vi "Gas_Setup.vi"() -> ()   [LabVIEW 2022 SP3]
uses:
  ADAM Controls/Ch_description_ADAM.ctl
  ADAM Controls/Module_type_ADAM.ctl
  ADAM Controls/Function_ADAM.ctl
  ADAM Controls/Channel_State.ctl
  ADAM Controls/Calib_type_ADAM.ctl
  ADAM Controls/Address.ctl
  ADAM Controls/Shut_Off_Valve.ctl
  ADAM Controls/Channel_names.ctl
  Channel_State_Control.ctl
  ADAM Controls/Update_scan_value.ctl
  Anemometry/Anemometry Sub Vis/Globals/Preference_global.vi
panel:
  in  "Change? 2":bool
  out "GMU2 Release Temp Channel":string
  in  "Change?":bool
  out "GMU1 Release Temp Channel":string
  out "Ch names":string[](array[string])
  in  "Select Plug Ins":bool
  in  "Source Info":string[][](table)
  in  "Carrier 1 Very Low":T1
  in  "Carrier 1 Hi-Tec Range":u16(ring) items=["Very Low", "High"]
  in  "Trace Hi-Tec Range":u16(ring) items=["25 ml/min", "300 ml/min"]
  in  "Carrier 1 High":T1
  in  "300 ml/min":T1
  in  "25 ml/min":T1
  in  "Release Orientation":u16(ring) items=["Vertical", "Horizontal 0 Deg", "Downwards", "External System Tests", "Horizontal", "Edit Strings"]
  in  "Source Type":u16(ring) items=["11mm downward facing", "1mm Annulus above tank wall with Internal 2mm Annulus floating roof at 50mm.", "2 x ID=11mm Holes", "23mm IDD=8mm", "2mm Annulus around a quarter of inside of tank wall", "2mm Annulus around inside of tank wall", "4 point source ID=8.5mm located 90 deg apart on 8cm Diameter", "4 x 3mm holes spaced 8mm apart at roof perimeter", "70x70mm", "8  x 3mm holes spaced 10mm apart at roof perimeter", "8mm Annulus around inside of tank wall", "B2 D=6.8mm", "B204 Height 244mm ID 5.5mm", "B230 Height 152.4mm ID 8.5mm", "B30 Area", "B311 ID=11mm", "B331 ID=5.4mm", "B38_8mm_ID_passive", "B38_OD=3.1mm_ID=2mm", "B548 OD=13.8mm ID=3.5mm", "Both_Scrubbers_ID=4mm", "Both_Scrubbers_ID=7mm", "Capped release D=10mm H=10mm Slot=2mm", "D=12mm", "D=13.6mm", "D=16mm (ID=12 mm)", "D=18mm", "D=20mm", "D=22.5mm", "D=3.4mm", "D=5mm (ground release)", "D=6mm (ID=4.2 mm)", "D=7.1mm", "D=9mm", "D=9mm  20mm long passive", "Dext = 8.5 mm", "Exit Port of Solenoid Valve", "H=25:W=100mm", "H=50", "ID=1.6 OD=1.9", "ID=1.9 OD=3.0mm", "ID=103mm", "ID=15 mm 90 deg bend copper tube", "ID=20mm", "ID=24mm", "ID=3.4mm  OD= 4mm", "ID=3.9mm OD=6.3mm", "ID=4.25mm", "ID=4mm", "ID=5.1mm OD=5.8mm (Ground release)", "ID=5.1mm OD=5.8mm (roof release)", "ID=5.1mm at Z= 10mm  (Ground release)", "ID=50mm", "ID=5mm OD=5.8mm", "ID=6mm", "ID=6mm OD=8mm", "ID=7.75mm OD=10mm", "ID=8.6mm", "ID=8mm OD=9mm", "ID=9.2mm", "ID=9.5mm OD=12.5mm", "ID=9mm OD=10mm  Short Passive", "Line Source 100mm  1.07m width", "Line Source 25mm  1.3m long  perp to flow", "Line Source 25x1300", "Line Source 50mm  1.07m Wide", "Line source parallel to flow", "None", "Permeability_rig", "Pond_No1&2_140mm", "Pond_No1&2_84mm", "Pond_No1_84mm", "Pond_No2_84mm", "ROSE 9mm at last grid", "SAV ID=3.5mm", "Sample tubes in source", "Single 5mm Stack", "Single 7.9 mm stack", "THORP  ID=5.1mm", "Twin 5mm Stacks", "Twin Passive Stacks ID=8mm OD=8.7mm", "UKAEA ID=1.7mm", "W=50mm", "Edit Strings"]
  in  "Gas Remaining":string[][](table)
  in  "Carrier 2 Gas":u16(ring) items=["Air", "Nitrogen", "Helium", "CO2", "Krypton", "None"]
  in  "Trace Gas":u16(ring) items=["Propane", "Ethane"]
  in  "Carrier 1 Gas":u16(ring) items=["Air", "Nitrogen", "Helium", "CO2", "Krypton", "None"]
  out "Numerical Values":dbl[](array[numeric]) format="%.9f"
  out "Ch Description Array":T2[](array[typedef]) {"Duty" format="%016b"; "D" format="%#_5g"; "C" format="%#_5g"; "B" format="%#_5g"; "A" format="%#_5g"}
  out "dup reference":refnum<vi>
  in  "stop":bool
  in  "OK":bool
  # "50l/min"
  # "50l/min"
  # "700l/min"
  # "50\nml/min"
  # "300\nml/min"
  # "5l/min"
  # "25\nml/min\nto Source"
  # "Very\nLow\nRange"
  # "High\nRange"
  # "Low\nRange"
  # "To Source"
  # "Dispersion Setup"
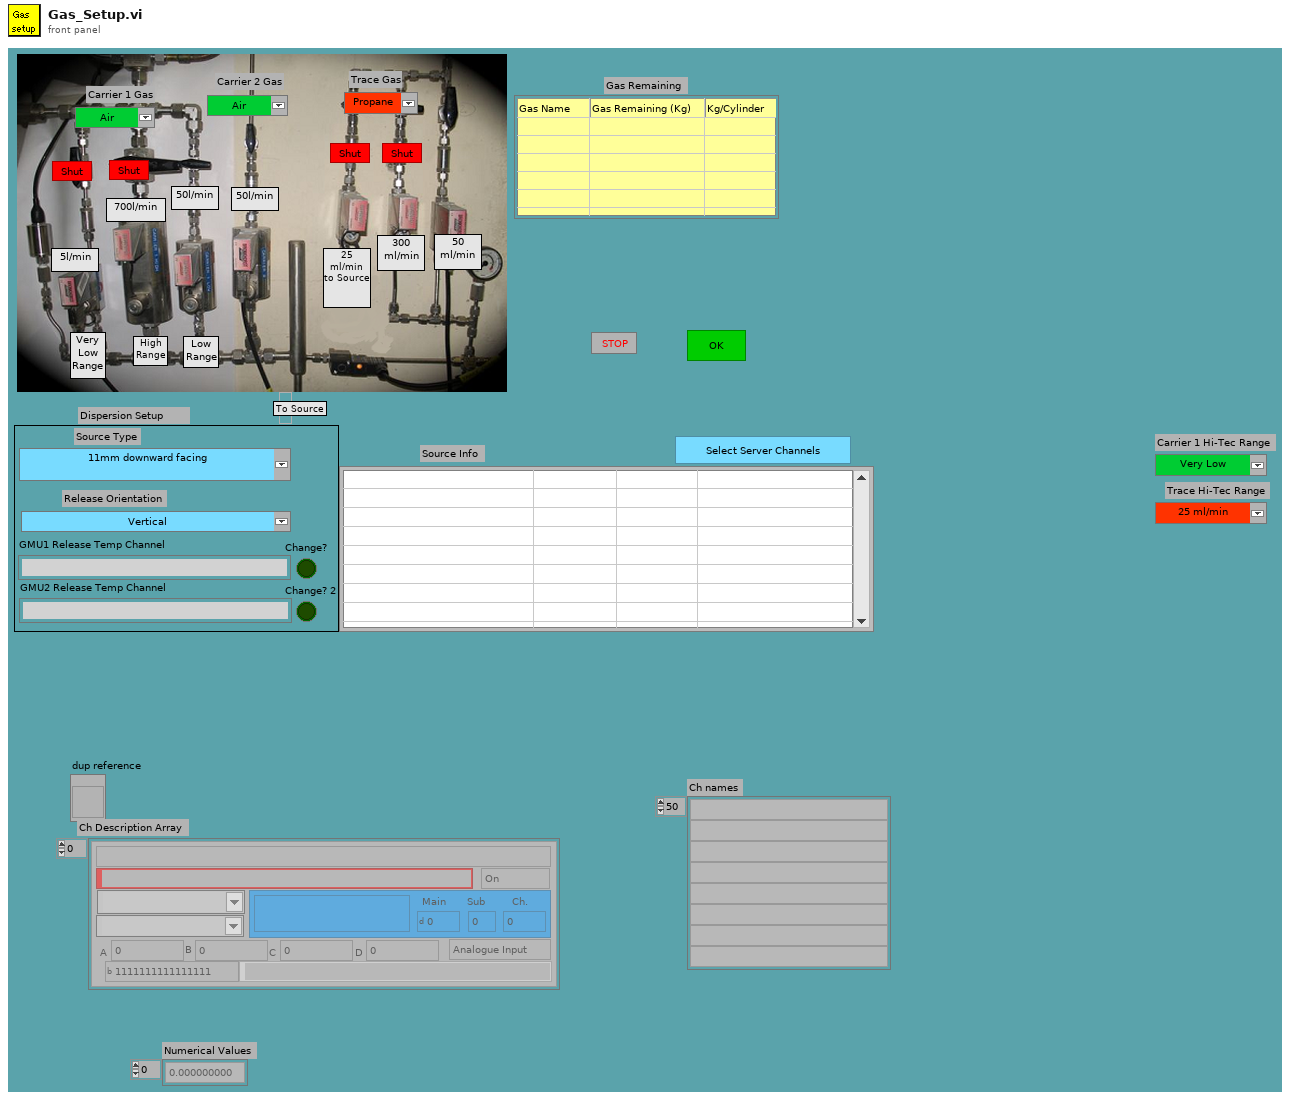
[diagram p1: front panel]
types:
  T1 = typedef "Shut_Off_Valve.ctl" = bool
  T2 = typedef "Ch_description_ADAM.ctl" = cluster{"Ch Name":string, "Type":T3, "Function":T4, "Ch State":T5, "Calibration type":T6, "A":dbl, "B":dbl, "C":dbl, "D":dbl, "Comments":string, "Address":T7, "String":string, "Duty":u16}
  T3 = typedef "Module_type_ADAM.ctl" = string
  T4 = typedef "Function_ADAM.ctl" = enum16{"Analogue Input", "Digital Input", "Event counter", "Event rate", "Analogue Output", "Digital Output", "Relay Output"}
  T5 = typedef "Channel_State.ctl" = enum16{"On", "Off", "Always On", "Always Off"}
  T6 = typedef "Calib_type_ADAM.ctl" = string
  T7 = typedef "Address.ctl" = cluster{"Main":i32, "Ch.":i32, "Sub":i32, "Port Name":string}
  T8 = typedef "Channel_names.ctl" = enum16{"Active Only", "Active + Off", "All Channels", "Changeable Only", "Always Off", "Always On", "Always Off or On"}
  T9 = typedef "Channel_State_Control.ctl" = enum16{"Channel Name", "Channel Name Starts with", "Main Address"}
  T10 = enum16{"Zero or one", "One", "Zero or more", "One or more"}
  T11 = typedef "Update_scan_value.ctl" = cluster{"Channel Name":string, "New Value":dbl, "!Auto_Off":bool}
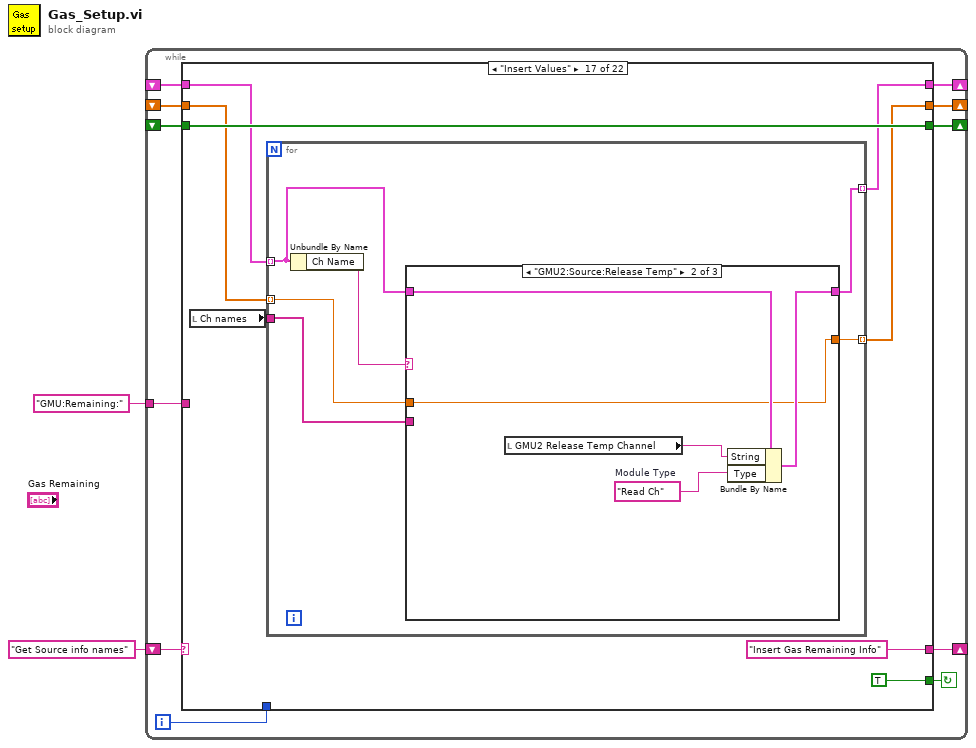
[diagram p0: block diagram]
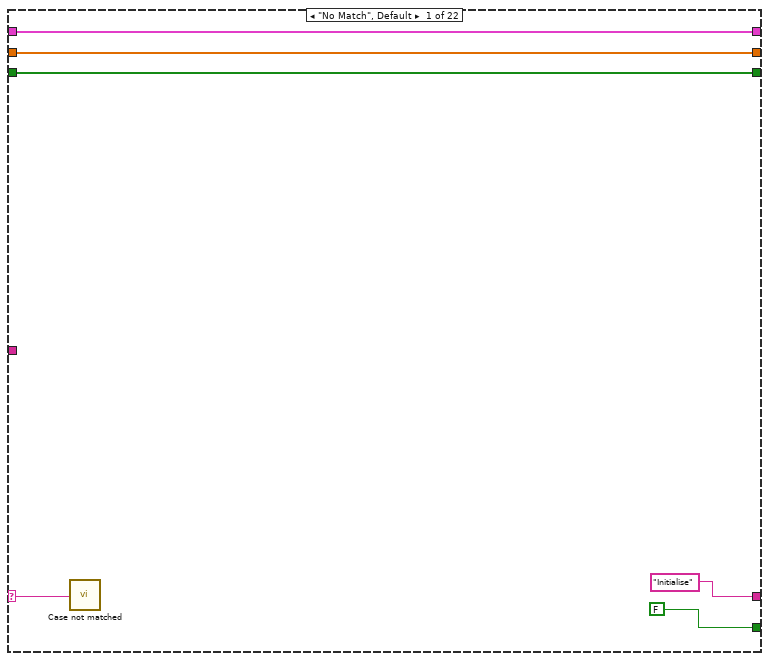
[diagram p2: hidden frame]
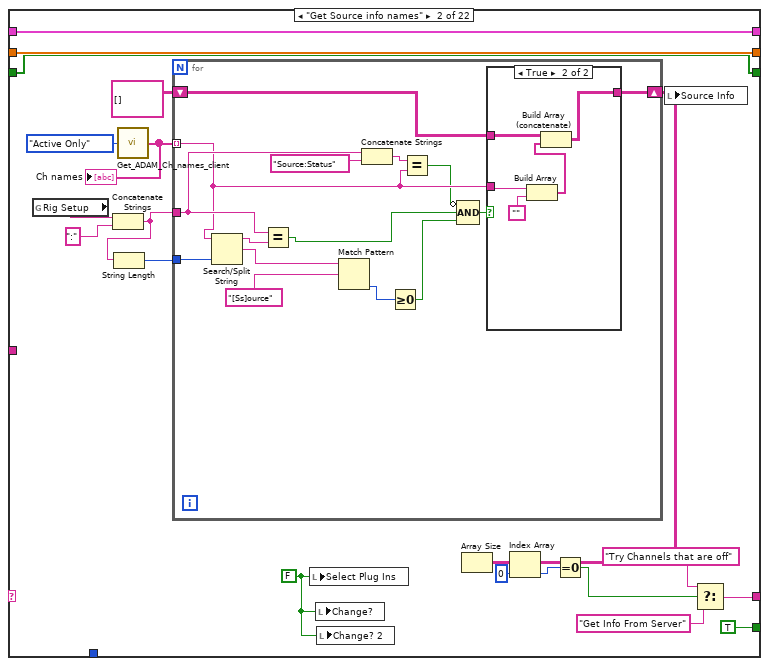
[diagram p3: hidden frame]
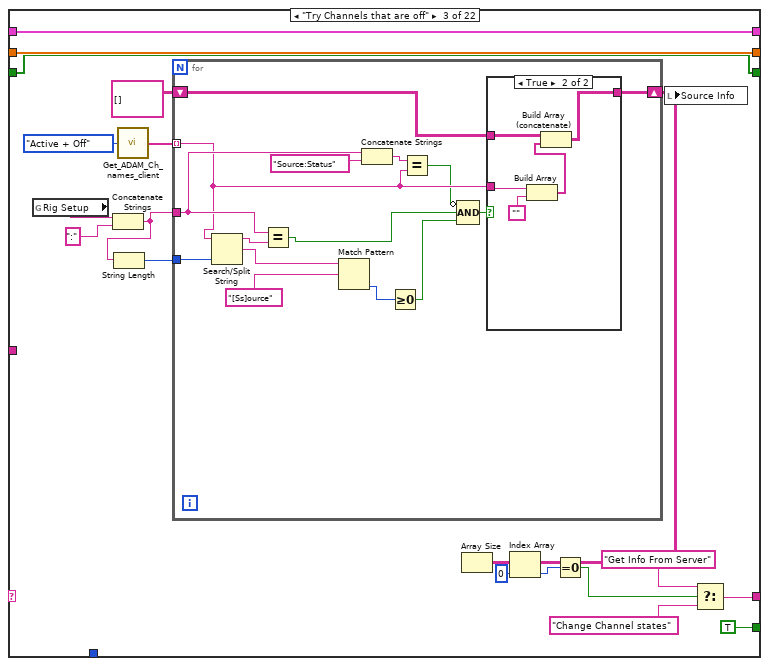
[diagram p5: hidden frame]
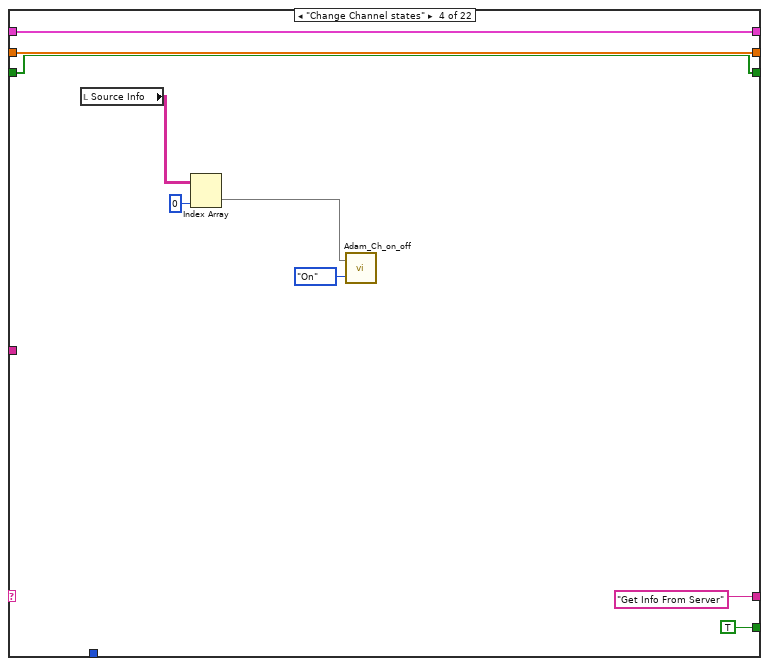
[diagram p7: hidden frame]
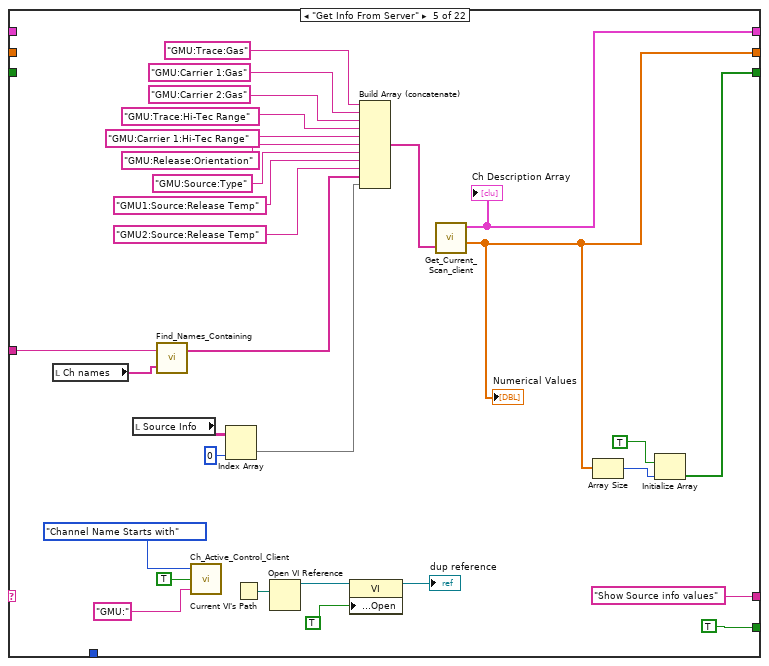
[diagram p8: hidden frame]
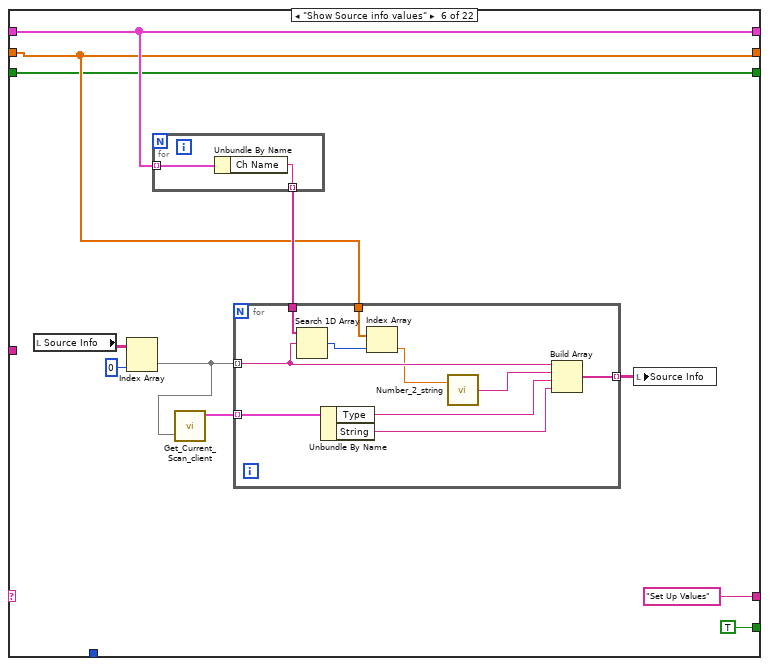
[diagram p9: hidden frame]
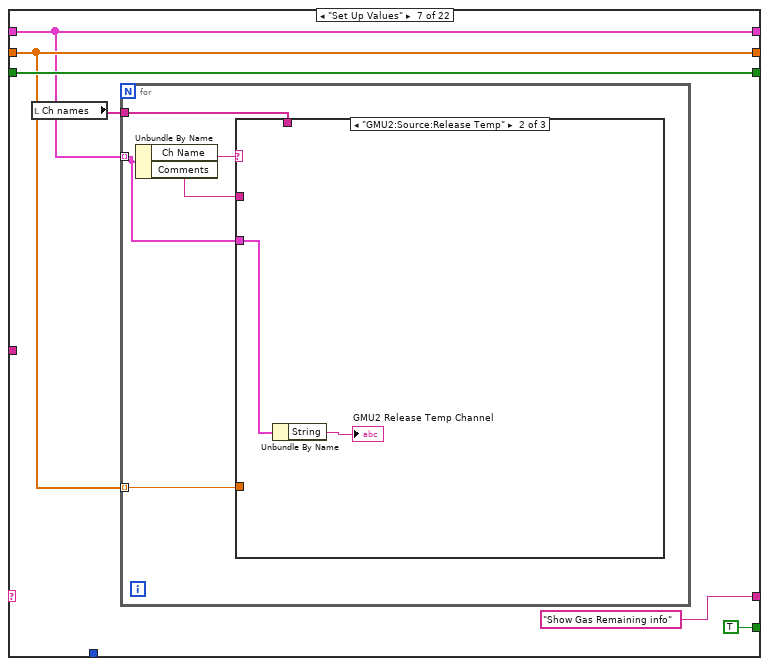
[diagram p10: hidden frame]
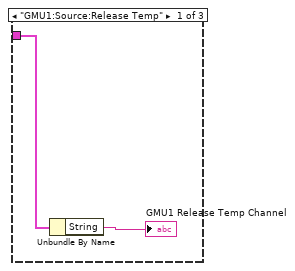
[diagram p11: hidden frame]
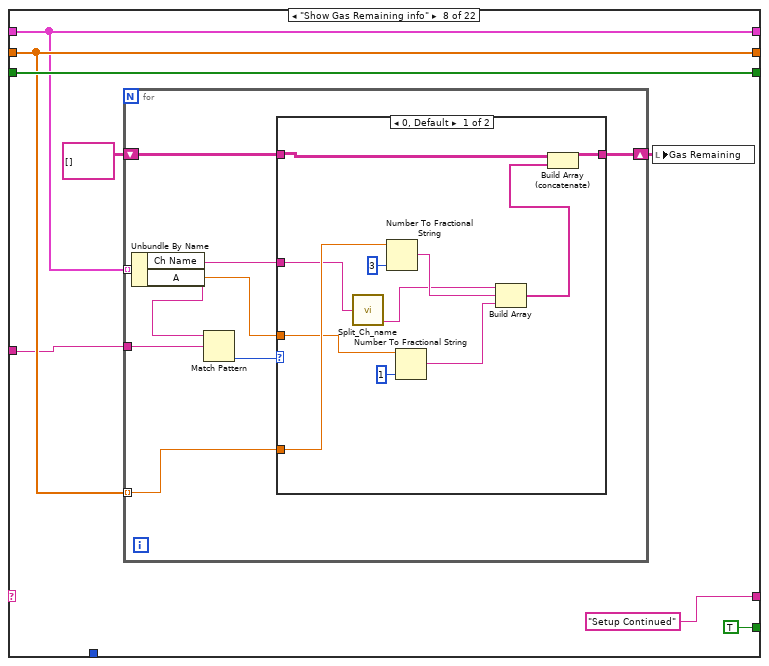
[diagram p13: hidden frame]
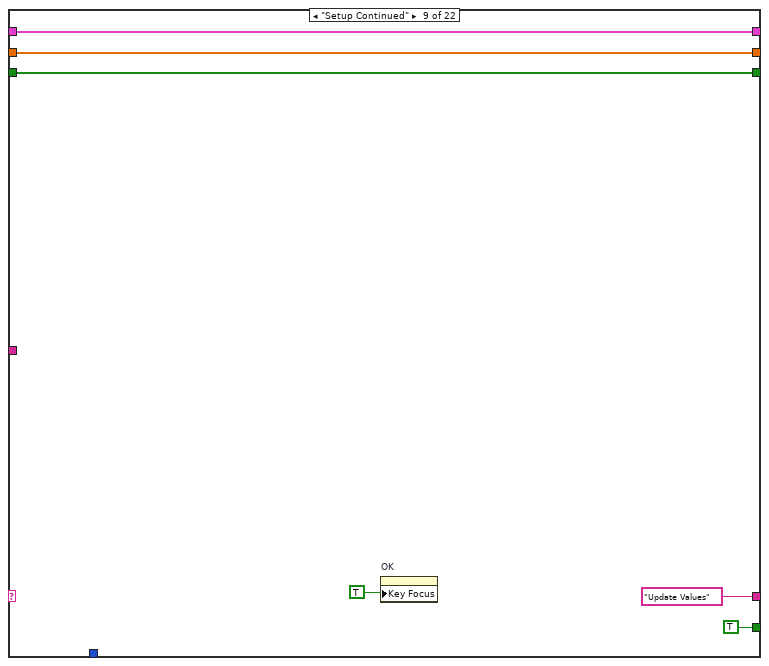
[diagram p15: hidden frame]
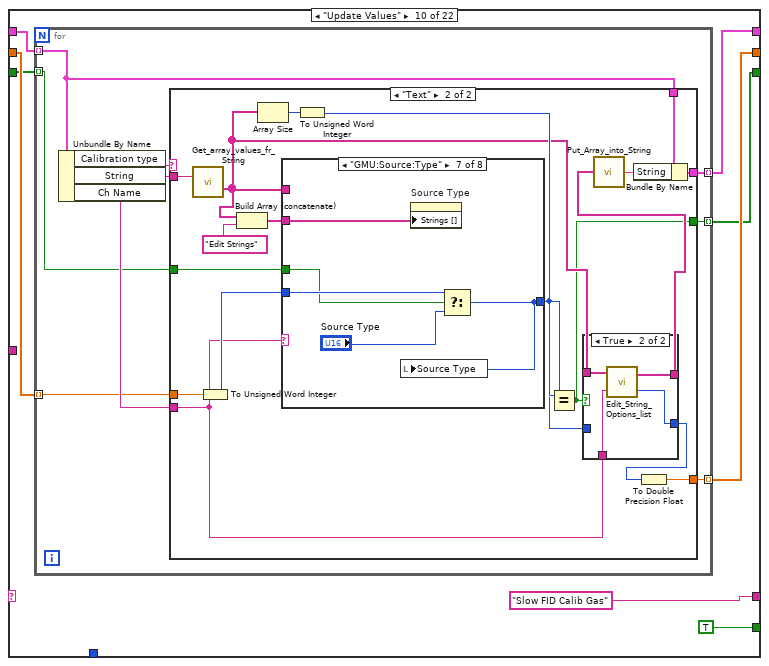
[diagram p16: hidden frame]
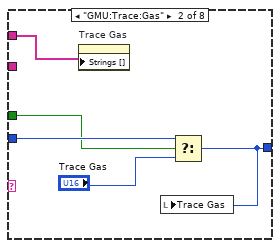
[diagram p20: hidden frame]
diagram:
  n1 = while {
    shift-left: _ -> [w5]
    shift-right: [w6] -> _
    shift-left: _ -> [w7]
    shift-right: [w9] -> _
    shift-left: _ -> [w8]
    shift-right: [w10] -> _
    shift-left: "Get Source info names" ("t") -> [w11]
    shift-right: [w12] -> _
    tunnel: "GMU:Remaining:" -> [w3]
    i -> [w4]
    stop <- w13 continue-if-true
    n2 = case shown="\"Insert Values\"" w11 {
      selector: w11 -> [w14 _ _ _ _ _ _ _ _ _ _ _ _ _ _ _ _ _ _ _ _ _]
      tunnel: [FALSE TRUE ("T button?") TRUE ("T button?") TRUE ("T button?") TRUE TRUE ("T button?") TRUE ("T button?") TRUE ("T button?") TRUE ("T button?") TRUE ("T button?") TRUE ("T button?") TRUE ("T button?") TRUE ("T button?") TRUE ("T button?") TRUE ("T button?") TRUE ("T button?") TRUE ("T button?") TRUE ("T button?") TRUE ("T button?") TRUE ("T button?") TRUE ("T button?") FALSE ("T button?")] -> w13
      tunnel: ["Initialise" w22 w63 "Get Info From Server" "Show Source info values" "Set Up Values" "Show Gas Remaining info" "Setup Continued" "Update Values" "Slow FID Calib Gas" w306 "Update Release Temperature" "Sort out Valve Logic" "Hi Tec Ranges" "Continue looping?" w411 "Insert Gas Remaining Info" "Insert Source info values" "Update Server" w498 "Get Source info names" ("t") "End"] -> w12
      tunnel: [w17 w35 w75 w109 w132 w149 w164 w181 w211 w217 w310 w339 w352 w357 w401 w417 w419 w447 w479 w507 w563 w614] -> w10
      tunnel: [w16 w34 w74 w108 w121 w148 w165 w182 w210 w215 w309 w338 w351 w356 w400 w416 w422 w453 w481 w506 w562 w613] -> w9
      tunnel: w8 -> [w17 w35 w75 w109 _ w149 w164 w181 w211 w218 w310 w339 w352 w357 w401 w417 w420 w447 w479 w507 w563 w614]
      tunnel: w7 -> [w16 w34 w74 w108 _ w148 w165 w182 w210 w216 w309 w338 w351 w356 w400 w416 w421 w452 w482 w506 w562 w613]
      tunnel: [w15 w33 w73 w107 w120 w147 w167 w184 w208 w212 w304 w336 w349 w354 w398 w410 w424 w455 w478 w505 w561 w606] -> w6
      tunnel: w5 -> [w15 w33 w73 w107 _ w147 w167 w184 w208 w213 w304 w336 w349 w354 w398 w410 w424 w455 w478 w505 w561 w606]
      tunnel: w4 -> [_ _ _ _ _ _ _ _ _ _ w303 _ _ _ _ _ _ _ _ _ _ _]
      tunnel: w3 -> [_ _ _ _ w118 _ _ w180 _ _ _ _ _ _ _ _ _ w446 _ _ _ _]
      frame "No Match", Default {
        n3 = call "Case not matched.vi"("Case Name not Matched"=w14) -> ()
      }
      frame "Get Source info names" {
        w20 = FALSE ("Select Plug Ins")
        n4 = global read "Preference_global.vi" "Rig Setup"() -> (w39:string)
        n5 = Concatenate Strings(w39, ":" ("string")) -> (w36:string)
        n6 = String Length(string=w36) -> (length=w37:i32)
        n7 = call "Get_ADAM_Ch_names_client.vi"("Channel names set"=Channel_names."Active Only") -> ("Ch names"=w30:string[])
        "Ch names" <- w30
        n8 = for {
          tunnel: w37 -> [w54]
          tunnel: w30 -> [w44] mode=indexing
          tunnel: w36 -> [w46]
          shift-right: [w48] -> w29
          shift-left: string[][] [] -> [w49]
          n9 = Search/Split String(string=w44, offset (0)=w54) -> (substring before match=w53:string, match + rest of string=w52:string)  [unwired: 2 out]
          n10 = Equal?(x=w46, y=w53) -> (x = y?=w42:bool)
          n11 = Match Pattern(string=w52, regular expression="[Ss]ource") -> (offset past match=w50:i32)  [unwired: 4 out]
          n12 = Concatenate Strings(w46, "Source:Status") -> (w45:string)
          n13 = Greater Or Equal To 0?(x=w50) -> (x >= 0?=w43:bool)
          n14 = Equal?(x=w45, y=w44) -> (x = y?=w41:bool)
          n15 = Compound Arithmetic op=AND(invert w41, w42, w43) -> (w40:bool)
          n16 = case shown="True" w40 {
            tunnel: w49 -> [w55 w60]
            tunnel: w44 -> [_ w58]
            tunnel: [w55 w59] -> w48
            frame False {
            }
            frame True {
              n17 = Build Array(w58, "") -> (w56:string[])
              n18 = Build Array (concatenate)(w60, w56) -> (w59:string[][])
            }
          }
        }
        n19 = local write "Select Plug Ins"(w20) -> ()
        n20 = local write "Change?"(w20) -> ()
        n21 = local write "Change? 2"(w20) -> ()
        n22 = Array Size(array=w29) -> (size(s)=w28:i32[])
        n23 = Index Array(array=w28, index=0) -> (element=w26:i32)
        n24 = Equal To 0?(x=w26) -> (x = 0?=w24:bool)
        n25 = local write "Source Info"(w29) -> ()
        n26 = Select(t="Try Channels that are off", s=w24, f="Get Info From Server") -> (s? t:f=w22:string)
      }
      frame "Try Channels that are off" {
        n27 = global read "Preference_global.vi" "Rig Setup"() -> (w79:string)
        n28 = Concatenate Strings(w79, ":" ("string")) -> (w76:string)
        n29 = String Length(string=w76) -> (length=w77:i32)
        n30 = call "Get_ADAM_Ch_names_client.vi"("Channel names set"=Channel_names."Active + Off") -> ("Ch names"=w70:string[])
        n31 = for {
          tunnel: w77 -> [w94]
          tunnel: w70 -> [w84] mode=indexing
          tunnel: w76 -> [w86]
          shift-right: [w88] -> w69
          shift-left: string[][] [] -> [w89]
          n32 = Search/Split String(string=w84, offset (0)=w94) -> (substring before match=w93:string, match + rest of string=w92:string)  [unwired: 2 out]
          n33 = Equal?(x=w86, y=w93) -> (x = y?=w82:bool)
          n34 = Match Pattern(string=w92, regular expression="[Ss]ource") -> (offset past match=w90:i32)  [unwired: 4 out]
          n35 = Concatenate Strings(w86, "Source:Status") -> (w85:string)
          n36 = Greater Or Equal To 0?(x=w90) -> (x >= 0?=w83:bool)
          n37 = Equal?(x=w85, y=w84) -> (x = y?=w81:bool)
          n38 = Compound Arithmetic op=AND(invert w81, w82, w83) -> (w80:bool)
          n39 = case shown="True" w80 {
            tunnel: w89 -> [w95 w100]
            tunnel: w84 -> [_ w98]
            tunnel: [w95 w99] -> w88
            frame False {
            }
            frame True {
              n40 = Build Array(w98, "") -> (w96:string[])
              n41 = Build Array (concatenate)(w100, w96) -> (w99:string[][])
            }
          }
        }
        n42 = Array Size(array=w69) -> (size(s)=w68:i32[])
        n43 = Index Array(array=w68, index=0) -> (element=w66:i32)
        n44 = Equal To 0?(x=w66) -> (x = 0?=w64:bool)
        n45 = local write "Source Info"(w69) -> ()
        n46 = Select(t="Get Info From Server", s=w64, f="Change Channel states") -> (s? t:f=w63:string)
      }
      frame "Change Channel states" {
        n47 = local read "Source Info"() -> (w104:string[][])
        n48 = Index Array(array=w104, index (col)=0 ("disabled index (col)")) -> (element=w102:string[])  [unwired: 1 in]
        n49 = call "Adam_Ch_on_off.vi"("Ch State"=Channel_State."On", "ADAM Ch Names"=w102) -> ()  [unwired: 1 out]
      }
      frame "Get Info From Server" {
        n50 = local read "Ch names"() -> (w111:string[])
        n51 = local read "Source Info"() -> (w114:string[][])
        n52 = call "Find_Names_Containing.vi"("Ch names"=w111, "String to match"=w118) -> ("Matched Names"=w119:string[])  [unwired: 1 out]
        n53 = call "Ch_Active_Control_Client.vi"("Match"="GMU:", "Activate Channels?"=TRUE, "Control on"=Channel_State_Control."Channel Name Starts with") -> ()  [unwired: 2 out]
        n54 = Index Array(array=w114, index (col)=0 ("disabled index (col)")) -> (element=w112:string[])  [unwired: 1 in]
        n55 = Current VI's Path() -> (path=w134:path)
        n56 = Open VI Reference(vi path=w134) -> (vi reference=w135:refnum<vi>)  [unwired: 1 in, 5 out]
        n57 = property class="VI"(reference=w135, "Front Panel Window:Open"=TRUE) -> (reference out=→"dup reference":refnum<vi>)  [unwired: 1 in, 1 out]
        n58 = Build Array (concatenate)("GMU:Trace:Gas", "GMU:Carrier 1:Gas", "GMU:Carrier 2:Gas", "GMU:Trace:Hi-Tec Range", "GMU:Carrier 1:Hi-Tec Range", "GMU:Release:Orientation", "GMU:Source:Type", "GMU1:Source:Release Temp", "GMU2:Source:Release Temp", w119, w112) -> (w137:string[])
        n59 = call "Get_Current_Scan_client.vi"("multipleChannels"=w137) -> ("Ch Description Array"=w132:T2[], "Numerical Values"=w121:dbl[])  [unwired: 1 in, 2 out]
        "Ch Description Array" <- w132
        "Numerical Values" <- w121
        n60 = Array Size(array=w121) -> (size(s)=w123:i32)
        n61 = Initialize Array(TRUE, w123) -> (w120:bool[])
      }
      frame "Show Source info values" {
        n62 = local read "Source Info"() -> (w143:string[][])
        n63 = Index Array(array=w143, index (col)=0 ("disabled index (col)")) -> (element=w141:string[])  [unwired: 1 in]
        n64 = for {
          tunnel: w149 -> [w162] mode=indexing
          tunnel: [w161] -> w150 mode=indexing
          n65 = Unbundle By Name(w162) -> ("Ch Name"=w161:string)
        }
        n66 = call "Get_Current_Scan_client.vi"("multipleChannels"=w141) -> ("Ch Description Array"=w140:T2[])  [unwired: 1 in, 3 out]
        n67 = for {
          tunnel: w150 -> [w160]
          tunnel: w141 -> [w157] mode=indexing
          tunnel: w148 -> [w158]
          tunnel: [w154] -> w146 mode=indexing
          tunnel: w140 -> [w153] mode=indexing
          n68 = Search 1D Array(1D array=w160, element=w157) -> (index of element=w159:i32)  [unwired: 1 out]
          n69 = Unbundle By Name(w153) -> ("Type"=w152:T3, "String"=w151:string)
          n70 = Index Array(array=w158, index=w159) -> (element=w156:dbl)
          n71 = call "Number_2_string.vi"("number"=w156) -> ("String"=w155:string)  [unwired: 1 in]
          n72 = Build Array(w157, w155, w152, w151) -> (w154:T3[])
        }
        n73 = local write "Source Info"(w146) -> ()
      }
      frame "Set Up Values" {
        n74 = local read "Ch names"() -> (w163:string[])
        n75 = for {
          tunnel: w165 -> [w169] mode=indexing
          tunnel: w164 -> [w171] mode=indexing
          tunnel: w163 -> [w170]
          n76 = Unbundle By Name(w171) -> ("Ch Name"=w173:string, "Comments"=w172:string)
          n77 = case shown="\"GMU2:Source:Release Temp\"" w173 {
            tunnel: w169 -> [_ _ _]
            tunnel: w172 -> [_ _ _]
            tunnel: w171 -> [w175 w177 _]
            tunnel: w170 -> [_ _ _]
            frame "GMU1:Source:Release Temp" {
              n78 = Unbundle By Name(w175) -> ("String"=→"GMU1 Release Temp Channel":string)
            }
            frame "GMU2:Source:Release Temp" {
              n79 = Unbundle By Name(w177) -> ("String"=→"GMU2 Release Temp Channel":string)
            }
            frame "No Match", Default {
            }
          }
        }
      }
      frame "Show Gas Remaining info" {
        n80 = for {
          tunnel: w182 -> [w188] mode=indexing
          tunnel: w181 -> [w193] mode=indexing
          tunnel: w180 -> [w192]
          shift-right: [w189] -> w178
          shift-left: string[][] [] -> [w190]
          n81 = Unbundle By Name(w193) -> ("Ch Name"=w186:string, "A"=w187:dbl)
          n82 = Match Pattern(string=w186, regular expression=w192) -> (offset past match=w191:i32)  [unwired: 4 out]
          n83 = case shown="0, Default" w191 {
            tunnel: w190 -> [w195 w205]
            tunnel: [w194 w205] -> w189
            tunnel: w188 -> [w199 _]
            tunnel: w187 -> [w198 _]
            tunnel: w186 -> [w197 _]
            frame 0, Default {
              n84 = call "Split_Ch_name.vi"("Ch name"=w197) -> ("Low level"=w201:string)  [unwired: 2 out]
              n85 = Number To Fractional String(number=w199, precision (6)=i16 3) -> (F-format string=w204:string)  [unwired: 2 out]
              n86 = Number To Fractional String(number=w198, precision (6)=i16 1) -> (F-format string=w202:string)  [unwired: 2 out]
              n87 = Build Array(w201, w204, w202) -> (w196:string[])
              n88 = Build Array (concatenate)(w195, w196) -> (w194:string[][])
            }
            frame -1 {
            }
          }
        }
        n89 = local write "Gas Remaining"(w178) -> ()
      }
      frame "Setup Continued" {
        n90 = property on="OK" class="Bool"("Key Focus"=TRUE ("Write Attribute")) -> ()  [unwired: 2 in, 2 out]
      }
      frame "Update Values" {
        n91 = for {
          tunnel: w218 -> [w225] mode=indexing
          tunnel: [w224] -> w217 mode=indexing
          tunnel: w216 -> [w223] mode=indexing
          tunnel: [w222] -> w215 mode=indexing
          tunnel: w213 -> [w221] mode=indexing
          tunnel: [w220] -> w212 mode=indexing
          n92 = Unbundle By Name(w225) -> ("Calibration type"=w228:T6, "String"=w227:string, "Ch Name"=w226:string)
          n93 = case shown="\"Text\"" w228 {
            tunnel: w227 -> [_ w249]
            tunnel: w226 -> [_ w239]
            tunnel: w225 -> [w231 w243]
            tunnel: [w231 w242] -> w224
            tunnel: w223 -> [w230 w241]
            tunnel: [w230 w240] -> w222
            tunnel: w221 -> [w229 w238]
            tunnel: [w229 w232] -> w220
            frame "Raw", Default {
            }
            frame "Text" {
              n94 = call "Get_array_values_fr_String.vi"("String Value"=w249) -> ("String array"=w236:string[])  [unwired: 1 out]
              n95 = To Unsigned Word Integer(number=w241) -> (unsigned 16bit integer=w247:u16)
              n96 = Build Array (concatenate)(w236, "Edit Strings") -> (w235:string[])
              n97 = Array Size(array=w236) -> (size(s)=w248:i32)
              n98 = case shown="\"GMU:Source:Type\"" w239 {
                tunnel: [w256 w260 w265 w270 w274 w278 w283 w288] -> w233
                tunnel: w236 -> [_ w258 w262 w268 _ _ _ _]
                tunnel: w247 -> [w256 w261 w266 w271 w275 w279 w284 w289]
                tunnel: w238 -> [_ w259 w264 w269 w273 w277 w282 w287]
                tunnel: w235 -> [_ _ _ _ _ _ w281 w286]
                frame "No match", Default {
                }
                frame "GMU:Trace:Gas" {
                  n99 = property on="Trace Gas" class="Ring (strict)"("Strings []"=w258) -> ()  [unwired: 2 in, 2 out]
                  n100 = Select(t=w261, s=w259, f="Trace Gas") -> (s? t:f=w260:u16)
                  n101 = local write "Trace Gas"(w260) -> ()
                }
                frame "GMU:Carrier 1:Gas" {
                  n102 = property on="Carrier 1 Gas" class="Ring (strict)"("Strings []"=w262) -> ()  [unwired: 2 in, 2 out]
                  n103 = Select(t=w266, s=w264, f="Carrier 1 Gas") -> (s? t:f=w265:u16)
                  n104 = local write "Carrier 1 Gas"(w265) -> ()
                }
                frame "GMU:Carrier 2:Gas" {
                  n105 = property on="Carrier 2 Gas" class="Ring (strict)"("Strings []"=w268) -> ()  [unwired: 2 in, 2 out]
                  n106 = Select(t=w271, s=w269, f="Carrier 2 Gas") -> (s? t:f=w270:u16)
                  n107 = local write "Carrier 2 Gas"(w270) -> ()
                }
                frame "GMU:Carrier 1:Hi-Tec Range" {
                  n108 = Select(t=w275, s=w273, f="Carrier 1 Hi-Tec Range") -> (s? t:f=w274:u16)
                  n109 = local write "Carrier 1 Hi-Tec Range"(w274) -> ()
                }
                frame "GMU:Trace:Hi-Tec Range" {
                  n110 = Select(t=w279, s=w277, f="Trace Hi-Tec Range") -> (s? t:f=w278:u16)
                  n111 = local write "Trace Hi-Tec Range"(w278) -> ()
                }
                frame "GMU:Source:Type" {
                  n112 = property on="Source Type" class="Ring (strict)"("Strings []"=w281) -> ()  [unwired: 2 in, 2 out]
                  n113 = Select(t=w284, s=w282, f="Source Type") -> (s? t:f=w283:u16)
                  n114 = local write "Source Type"(w283) -> ()
                }
                frame "GMU:Release:Orientation" {
                  n115 = property on="Release Orientation" class="Ring (strict)"("Strings []"=w286) -> ()  [unwired: 2 in, 2 out]
                  n116 = Select(t=w289, s=w287, f="Release Orientation") -> (s? t:f=w288:u16)
                  n117 = local write "Release Orientation"(w288) -> ()
                }
              }
              n118 = To Unsigned Word Integer(number=w248) -> (unsigned 16bit integer=w246:u16)
              n119 = Equal?(x=w246, y=w233) -> (x = y?=w232:bool)
              n120 = case shown="True" w232 {
                tunnel: w236 -> [w251 w255]
                tunnel: w239 -> [_ w254]
                tunnel: [w251 w253] -> w244
                tunnel: [w250 w252] -> w234
                tunnel: w233 -> [w250 _]
                frame False {
                }
                frame True {
                  n121 = call "Edit_String_Options_list.vi"("Channel Name"=w254, "String array"=w255) -> ("New Selection Index"=w252:i32, "String array Out"=w253:string[])
                }
              }
              n122 = call "Put_Array_into_String.vi"("String array"=w244) -> ("String Value"=w245:string)
              n123 = Bundle By Name(cluster=w243, "String"=w245) -> (w242:T2)
              n124 = To Double Precision Float(number=w234) -> (double precision float=w240:dbl)
            }
          }
        }
      }
      frame "Slow FID Calib Gas" {
        n125 = local read "Ch names"() -> (w291:string[])
        n126 = local read "GMU1 Release Temp Channel"() -> (w296:string)
        n127 = local read "GMU2 Release Temp Channel"() -> (w295:string)
        n128 = Less?(x=w303, y=10) -> (x < y?=w301:bool)
        n129 = Search 1D Array(1D array=w291, element=w296) -> (index of element=w300:i32)  [unwired: 1 in]
        n130 = Search 1D Array(1D array=w291, element=w295) -> (index of element=w292:i32)  [unwired: 1 in]
        n131 = Less Than 0?(x=w300) -> (x < 0?=w299:bool)
        n132 = Less Than 0?(x=w292) -> (x < 0?=w293:bool)
        n133 = Or(x=w299, y="Change?") -> (x .or. y?=w298:bool)
        n134 = Or(x=w293, y="Change? 2") -> (x .or. y?=w294:bool)
        n135 = case shown="True" w298 {
          tunnel: w291 -> [_ w328]
          tunnel: w296 -> [_ w326]
          frame False {
          }
          frame True {
            n136 = Build Array(w326) -> (w325:string[])
            n137 = call "Select_Strings.vi"("Timeout (s)"=nan, "Available Ch names"=w328, "Message"="Please choose the Reference Temperature for GMU1", "Selector mode"=T10."One", "Desired Ch names (in)"=w325) -> ("Selected Channel Names"=w321:string[])  [unwired: 1 in, 2 out]
            n138 = Index Array(array=w321) -> (element=w320:string)  [unwired: 1 in]
            n139 = local write "GMU1 Release Temp Channel"(w320) -> ()
            n140 = local write "Change?"(FALSE ("Change?")) -> ()
          }
        }
        n141 = case shown="True" w294 {
          tunnel: w291 -> [_ w319]
          tunnel: w295 -> [_ w317]
          frame False {
          }
          frame True {
            n142 = Build Array(w317) -> (w316:string[])
            n143 = call "Select_Strings.vi"("Timeout (s)"=nan, "Available Ch names"=w319, "Message"="Please choose the Reference Temperature for GMU2", "Selector mode"=T10."One", "Desired Ch names (in)"=w316) -> ("Selected Channel Names"=w312:string[])  [unwired: 1 in, 2 out]
            n144 = Index Array(array=w312) -> (element=w311:string)  [unwired: 1 in]
            n145 = local write "GMU2 Release Temp Channel"(w311) -> ()
            n146 = local write "Change? 2"(FALSE ("Change?")) -> ()
          }
        }
        n147 = Select(t="Initialise Hi tec selection", s=w301, f="Update Release Temperature") -> (s? t:f=w306:string)
      }
      frame "Initialise Hi tec selection" {
        n148 = local read "Carrier 1 Hi-Tec Range"() -> (w334:u16)
        n149 = local read "Trace Hi-Tec Range"() -> (w331:u16)
        n150 = case shown="1" w334 {
          tunnel: [FALSE TRUE] -> w333
          tunnel: [TRUE FALSE] -> w332
          frame 0, Default {
          }
          frame 1 {
          }
        }
        n151 = case shown="1" w331 {
          tunnel: [TRUE FALSE] -> w330
          tunnel: [FALSE TRUE] -> w329
          frame 0, Default {
          }
          frame 1 {
          }
        }
        n152 = local write "Carrier 1 Very Low"(w332) -> ()
        n153 = local write "Carrier 1 High"(w333) -> ()
        n154 = local write "25 ml/min"(w330) -> ()
        n155 = local write "300 ml/min"(w329) -> ()
      }
      frame "Update Release Temperature" {
      }
      frame "Sort out Valve Logic" {
        n156 = while {
          shift-left: _ -> [w359]
          shift-right: [w360] -> _
          shift-left: _ -> [w361]
          shift-right: [w364] -> _
          shift-left: _ -> [w362]
          shift-right: [w363] -> _
          shift-left: _ -> [w365]
          shift-right: [w366] -> _
          stop <- FALSE continue-if-true
          n157 = stacked-sequence {
            tunnel: ["Carrier 1 High" _] -> w366
            tunnel: w365 -> [w373 _]
            tunnel: [_ "300 ml/min"] -> w364
            tunnel: [_ "25 ml/min"] -> w363
            tunnel: w362 -> [_ w383]
            tunnel: w361 -> [_ w382]
            tunnel: ["Carrier 1 Very Low" _] -> w360
            tunnel: w359 -> [w368 _]
            frame #0 {
              n158 = Build Array("Carrier 1 Very Low", "Carrier 1 High") -> (w372:T1[])
              n159 = Boolean To (0,1)(Boolean=w372) -> (0, 1=w371:i16[])
              n160 = Add Array Elements(numeric array=w371) -> (sum=w370:i16)
              n161 = case shown="2, Default" w370 {
                tunnel: w373 -> [_ _ w377]
                tunnel: "Carrier 1 Very Low" -> [_ _ w379]
                tunnel: w368 -> [_ _ w378]
                tunnel: "Carrier 1 High" -> [_ _ w376]
                frame 0 {
                }
                frame 1 {
                }
                frame 2, Default {
                  n162 = Exclusive Or(1:w378, 2:w379) -> (0:w375:T1)
                  n163 = Exclusive Or(1:w377, 2:w376) -> (0:w374:T1)
                  n164 = local write "Carrier 1 Very Low"(w375) -> ()
                  n165 = local write "Carrier 1 High"(w374) -> ()
                }
              }
            }
            frame #1 {
              n166 = Build Array("25 ml/min", "300 ml/min") -> (w386:T1[])
              n167 = Boolean To (0,1)(Boolean=w386) -> (0, 1=w385:i16[])
              n168 = Add Array Elements(numeric array=w385) -> (sum=w384:i16)
              n169 = case shown="2, Default" w384 {
                tunnel: w383 -> [_ _ w392]
                tunnel: w382 -> [_ _ w391]
                tunnel: "300 ml/min" -> [_ _ w390]
                tunnel: "25 ml/min" -> [_ _ w389]
                frame 0 {
                }
                frame 1 {
                }
                frame 2, Default {
                  n170 = Exclusive Or(1:w391, 2:w390) -> (0:w387:T1)
                  n171 = Exclusive Or(1:w392, 2:w389) -> (0:w388:T1)
                  n172 = local write "300 ml/min"(w387) -> ()
                  n173 = local write "25 ml/min"(w388) -> ()
                }
              }
            }
          }
        }
      }
      frame "Hi Tec Ranges" {
        n174 = local read "Carrier 1 Very Low"() -> (w394:T1)
        n175 = local read "25 ml/min"() -> (w395:T1)
        n176 = case shown="False" w394 {
          tunnel: [u16 1 ("Carrier 1 Hi-Tec Range") u16 0 ("Carrier 1 Hi-Tec Range")] -> w393
          frame False {
          }
          frame True {
          }
        }
        n177 = case shown="False" w395 {
          tunnel: [u16 1 ("Carrier 1 Hi-Tec Range") u16 0 ("Carrier 1 Hi-Tec Range")] -> w396
          frame False {
          }
          frame True {
          }
        }
        n178 = local write "Carrier 1 Hi-Tec Range"(w393) -> ()
        n179 = local write "Trace Hi-Tec Range"(w396) -> ()
      }
      frame "Continue looping?" {
        n180 = local read "Select Plug Ins"() -> (w407:bool)
        n181 = Compound Arithmetic op=OR("stop", "OK", w407) -> (w406:bool)
        n182 = Current VI's Path() -> (path=w414:path)
        n183 = call "Close_Panel_and_Abort.vi"("Vi path"=w414, "stop"="stop") -> ()  [unwired: 1 out]
        n184 = Select(t="Insert Values", s=w406, f="Update Values") -> (s? t:f=w411:string)
      }
      frame "Insert Values" {
        n185 = local read "Ch names"() -> (w418:string[])
        n186 = for {
          tunnel: w420 -> [w428] mode=indexing
          tunnel: w421 -> [w430] mode=indexing
          tunnel: [w429] -> w422 mode=indexing
          tunnel: [w427] -> w419 mode=indexing
          tunnel: w418 -> [w426]
          n187 = Unbundle By Name(w428) -> ("Ch Name"=w431:string)
          n188 = case shown="\"GMU2:Source:Release Temp\"" w431 {
            tunnel: w430 -> [w432 w437 w443]
            tunnel: [w432 w437 w443] -> w429
            tunnel: w428 -> [w435 w440 w442]
            tunnel: [w434 w439 w442] -> w427
            tunnel: w426 -> [_ _ _]
            frame "GMU1:Source:Release Temp" {
              w436 = T3 "Read Ch"  # Module Type
              n189 = local read "GMU1 Release Temp Channel"() -> (w433:string)
              n190 = Bundle By Name(cluster=w435, "String"=w433, "Type"=w436) -> (w434:T2)
            }
            frame "GMU2:Source:Release Temp" {
              w441 = T3 "Read Ch"  # Module Type
              n191 = local read "GMU2 Release Temp Channel"() -> (w438:string)
              n192 = Bundle By Name(cluster=w440, "String"=w438, "Type"=w441) -> (w439:T2)
            }
            frame "No Match", Default {
            }
          }
        }
      }
      frame "Insert Gas Remaining Info" {
        n193 = local read "Gas Remaining"() -> (w449:string[][])
        n194 = Index Array(array=w449, index (col)=0 ("disabled index (col)")) -> (element=w445:string[])  [unwired: 1 in]
        n195 = for {
          tunnel: w446 -> [w459]
          tunnel: w445 -> [w458] mode=indexing
          tunnel: [w457] -> w444 mode=indexing
          n196 = Concatenate Strings(w459, w458) -> (w457:string)
        }
        n197 = Index Array(array=w449, index (col)=1 ("disabled index (col)")) -> (element=w448:string[])  [unwired: 1 in]
        n198 = for {
          tunnel: w447 -> [w472] mode=indexing
          tunnel: w452 -> [w460] mode=indexing
          tunnel: [w468] -> w453 mode=indexing
          tunnel: w444 -> [w471]
          tunnel: w448 -> [w469]
          n199 = Unbundle By Name(w472) -> ("Ch Name"=w470:string)
          n200 = Search 1D Array(1D array=w471, element=w470) -> (index of element=w466:i32)  [unwired: 1 out]
          n201 = Number To Fractional String(number=w460, precision (6)=i16 3) -> (F-format string=w464:string)  [unwired: 2 out]
          n202 = Index Array(array=w469, index=w466) -> (element=w465:string)
          n203 = Greater Or Equal To 0?(x=w466) -> (x >= 0?=w463:bool)
          n204 = Not Equal?(x=w464, y=w465) -> (x != y?=w462:bool)
          n205 = And(x=w462, y=w463) -> (x .and. y?=w461:bool)
          n206 = case shown="False" w461 {
            tunnel: [w473 w475] -> w468
            tunnel: w465 -> [_ w474]
            tunnel: w460 -> [w473 _]
            frame False {
            }
            frame True {
              n207 = Fract/Exp String To Number(string=w474) -> (number=w475:dbl)  [unwired: 4 out]
            }
          }
        }
      }
      frame "Insert Source info values" {
        n208 = for {
          tunnel: w479 -> [w496] mode=indexing
          tunnel: [w495] -> w487 mode=indexing
          n209 = Unbundle By Name(w496) -> ("Ch Name"=w495:string)
        }
        n210 = Index Array(array="Source Info", index (col)=0 ("disabled index (col)")) -> (element=w483:string[])  [unwired: 1 in]
        n211 = Index Array(array="Source Info", index (col)=1 ("disabled index (col)")) -> (element=w480:string[])  [unwired: 1 in]
        n212 = for {
          tunnel: w487 -> [w494]
          tunnel: w483 -> [w493] mode=indexing
          shift-right: [w490] -> w481
          shift-left: w482 -> [w491]
          tunnel: w480 -> [w489] mode=indexing
          n213 = Fract/Exp String To Number(string=w489) -> (number=w488:dbl)  [unwired: 4 out]
          n214 = Search 1D Array(1D array=w494, element=w493) -> (index of element=w492:i32)  [unwired: 1 out]
          n215 = Replace Array Subset(array=w491, new element=w488, index=w492) -> (w490:dbl[])
        }
      }
      frame "Update Server" {
        w502 = T11 {"Channel Name"="", "New Value"=0.0, "!Auto_Off"=FALSE} ("Update Scan Value Cluster")
        n216 = Index Array(array=w507, index=0 ("Index")) -> (element=w518:T2)
        n217 = local read "Ch Description Array"() -> (w504:T2[])
        n218 = local read "Numerical Values"() -> (w503:dbl[])
        n219 = Initialize Array(w518, 0 ("Dimension Size")) -> (w516:T2[])
        n220 = Initialize Array(w502, 0 ("Dimension Size")) -> (w511:T11[])
        n221 = for {
          shift-right: [w531] -> w513
          shift-left: w516 -> [w532]
          tunnel: w507 -> [w522] mode=indexing
          shift-right: [w530] -> w508
          shift-left: w511 -> [w529]
          tunnel: w506 -> [w524] mode=indexing
          tunnel: w504 -> [w523] mode=indexing
          tunnel: w503 -> [w527] mode=indexing
          tunnel: w502 -> [w525]
          n222 = Equal?(x=w522, y=w523) -> (x = y?=w528:bool)
          n223 = Equal?(x=w524, y=w527) -> (x = y?=w526:bool)
          n224 = case shown="False" w526 {
            tunnel: w529 -> [w539 w540]
            tunnel: [w538 w540] -> w530
            tunnel: w525 -> [w537 _]
            tunnel: w524 -> [w536 _]
            tunnel: w522 -> [w535 _]
            frame False {
              n225 = Unbundle By Name(w535) -> ("Ch Name"=w534:string)
              n226 = Bundle By Name(cluster=w537, "Channel Name"=w534, "New Value"=w536) -> (w533:T11)
              n227 = Build Array (concatenate)(w539, w533) -> (w538:T11[])
            }
            frame True {
            }
          }
          n228 = case shown="False" w528 {
            tunnel: w532 -> [w543 w544]
            tunnel: w522 -> [w542 _]
            tunnel: [w541 w544] -> w531
            frame False {
              n229 = Build Array (concatenate)(w543, w542) -> (w541:T2[])
            }
            frame True {
            }
          }
        }
        n230 = Array Size(array=w513) -> (size(s)=w515:i32)
        n231 = Array Size(array=w508) -> (size(s)=w509:i32)
        n232 = Greater Than 0?(x=w515) -> (x > 0?=w514:bool)
        n233 = Greater Than 0?(x=w509) -> (x > 0?=w510:bool)
        n234 = case shown="True" w514 {
          tunnel: w513 -> [_ w521]
          frame False {
          }
          frame True {
            n235 = call "Update_Ch_Discription_client.vi"("Channels to update In"=w521) -> ()  [unwired: 1 out]
          }
        }
        n236 = case shown="True" w510 {
          tunnel: w508 -> [_ w520]
          frame False {
          }
          frame True {
            n237 = call "Update_Current_Value_client.vi"("Update array in"=w520) -> ()  [unwired: 1 in]
          }
        }
        n238 = Select(t="Select Server Channels", s="Select Plug Ins", f="Close Panel") -> (s? t:f=w498:string)
      }
      frame "Select Server Channels" {
        w548 = string[] []
        w557 = T10."Zero or more"  # Selector mode
        n239 = local read "Source Info"() -> (w555:string[][])
        n240 = global read "Preference_global.vi" "Rig Setup"() -> (w568:string)
        n241 = Concatenate Strings(w568, ":" ("string")) -> (w565:string)
        n242 = String Length(string=w565) -> (length=w566:i32)
        n243 = call "Get_ADAM_Ch_names_client.vi"("Channel names set"=Channel_names."All Channels") -> ("Ch names"=w558:string[])
        n244 = Index Array(array=w555, index (col)=0) -> (element=w550:string[])  [unwired: 1 in]
        n245 = for {
          tunnel: w566 -> [w601]
          tunnel: w558 -> [w591] mode=indexing
          tunnel: w565 -> [w593]
          shift-right: [w595] -> w556
          shift-left: string[] [] -> [w596]
          n246 = Search/Split String(string=w591, offset (0)=w601) -> (substring before match=w600:string, match + rest of string=w599:string)  [unwired: 2 out]
          n247 = Equal?(x=w593, y=w600) -> (x = y?=w589:bool)
          n248 = Match Pattern(string=w599, regular expression="[Ss]ource") -> (offset past match=w597:i32)  [unwired: 4 out]
          n249 = Concatenate Strings(w593, "Source:Status") -> (w592:string)
          n250 = Greater Or Equal To 0?(x=w597) -> (x >= 0?=w590:bool)
          n251 = Equal?(x=w592, y=w591) -> (x = y?=w588:bool)
          n252 = Compound Arithmetic op=AND(invert w588, w589, w590) -> (w587:bool)
          n253 = case shown="True" w587 {
            tunnel: w596 -> [w602 w605]
            tunnel: w591 -> [_ w603]
            tunnel: [w602 w604] -> w595
            frame False {
            }
            frame True {
              n254 = Build Array (concatenate)(w605, w603) -> (w604:string[])
            }
          }
        }
        n255 = call "Select_Strings.vi"("Available Ch names"=w556, "Message"="Please select the appropriate source information channels", "Selector mode"=w557, "Desired Ch names (in)"=w550) -> ("Selected Channel Names"=w549:string[])  [unwired: 1 in, 3 out]
        n256 = for {
          tunnel: w550 -> [w572] mode=indexing
          tunnel: w549 -> [w573]
          shift-right: [w569] -> w547
          shift-left: w548 -> [w570]
          n257 = Search 1D Array(1D array=w573, element=w572) -> (index of element=w571:i32)  [unwired: 1 out]
          n258 = case shown="-1" w571 {
            tunnel: w572 -> [_ w577]
            tunnel: w570 -> [w574 w576]
            tunnel: [w574 w575] -> w569
            frame 0, Default {
            }
            frame -1 {
              n259 = Build Array (concatenate)(w576, w577) -> (w575:string[])
            }
          }
        }
        n260 = call "Adam_Ch_on_off.vi"("Ch State"=Channel_State."Always Off", "ADAM Ch Names"=w547) -> ()  [unwired: 1 out]
        n261 = for {
          tunnel: w549 -> [w581] mode=indexing
          tunnel: w550 -> [w582]
          shift-right: [w578] -> w551
          shift-left: w548 -> [w579]
          n262 = Search 1D Array(1D array=w582, element=w581) -> (index of element=w580:i32)  [unwired: 1 out]
          n263 = case shown="-1" w580 {
            tunnel: w581 -> [_ w586]
            tunnel: w579 -> [w583 w585]
            tunnel: [w583 w584] -> w578
            frame 0, Default {
            }
            frame -1 {
              n264 = Build Array (concatenate)(w585, w586) -> (w584:string[])
            }
          }
        }
        n265 = call "Adam_Ch_on_off.vi"("Ch State"=Channel_State."On", "ADAM Ch Names"=w551) -> ()  [unwired: 1 out]
      }
      frame "Close Panel" {
        n266 = local read "dup reference"() -> (w607:refnum<vi>)
        n267 = property class="VI"(reference=w607, "Front Panel Window:Open"=FALSE) -> (reference out=w609:refnum<vi>, error out=w608:errorcluster)  [unwired: 1 in]
        n268 = Close Reference(reference=w609, error in (no error)=w608) -> ()  [unwired: 1 out]
      }
    }
  }
